vi "BG2FGV.vi"(8 "Error In":errorcluster, 10 "action":enum16{"write", "read"}(ring)=enum."read", 11 "BG2 in":dbl[](array[numeric])) -> (0 "Error Out":errorcluster, 3 "BG2 out":dbl[](array[numeric]))   [LabVIEW 2020]
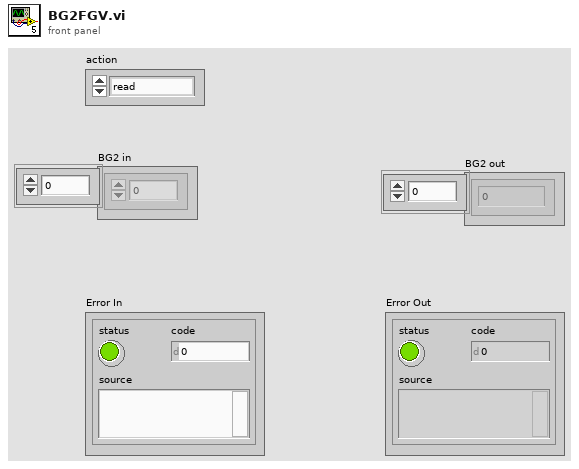
[diagram p1: front panel]
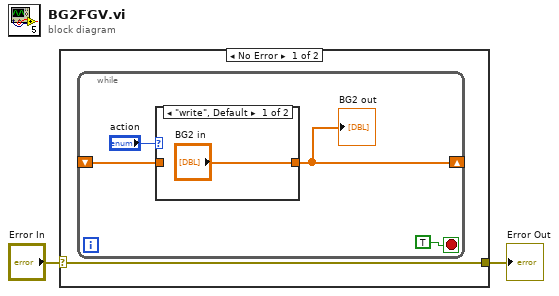
[diagram p0: block diagram]
diagram:
  n1 = case shown="No Error" "Error In" {
    selector: "Error In" -> [w3 w10]
    tunnel: [w3 w10] -> w1
    frame No Error {
      n2 = while {
        shift-right: [w6] -> _
        shift-left: _ -> [w4]
        stop <- TRUE stop-if-true
        n3 = case shown="\"write\", Default" "action" {
          tunnel: ["BG2 in" w9] -> w6
          tunnel: w4 -> [_ w9]
          frame "write", Default {
          }
          frame "read" {
          }
        }
        "BG2 out" <- w6
      }
    }
    frame Error {
    }
  }
  "Error Out" <- w1
